vi "Initialize.vi"(8 "error in (no error)":errorcluster, 10 "Pixel Mode (0:Optical)":u16(ring) items=["Optical ", "All Pixels"], 11 "VISA resource name":refnum<visa-resource-name>) -> (0 "error out":errorcluster, 3 "VISA resource name out":refnum<visa-resource-name>)   [LabVIEW 2019, in "Ocean Optics 2000 4000.lvlib"]
doc: "Establishes communication with the instrument and optionally performs an instrument identification query and/or an instrument reset. It also places the instrument in a default state needed for other instrument driver operations. Therefore, call this VI before calling other instrument driver VIs for this instrument. Generally, you need to call the Initialize VI only once at the beginning of an application."
uses:
  Ocean Optics 2000 4000.lvlib
panel:
  # "(c) 2009-2016 National Instruments.  ALL RIGHTS RESERVED."
  # "Before using this driver:\n    * Go to Program Files >>National Instruments >>LabVIEW >> \n       instr.lib>> Ocean Optics 2000 4000>>VISA_USB\n    * Select the folder for the model of instrument you are using.\n    * For Windows Vista, use the INF file with _vista in the file name\n      (eg.Ocean Optics USB4000_vista.inf). For XP, use the other INF file.\n    * To install, right click and select Install.\n    * NI MAX should be able to detect this instrument after installing the \n      INF file."
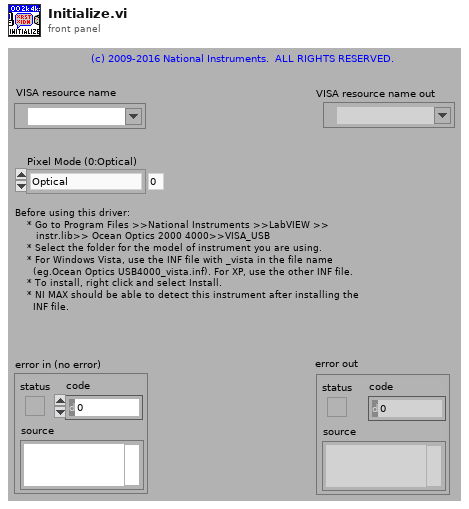
[diagram p1: front panel]
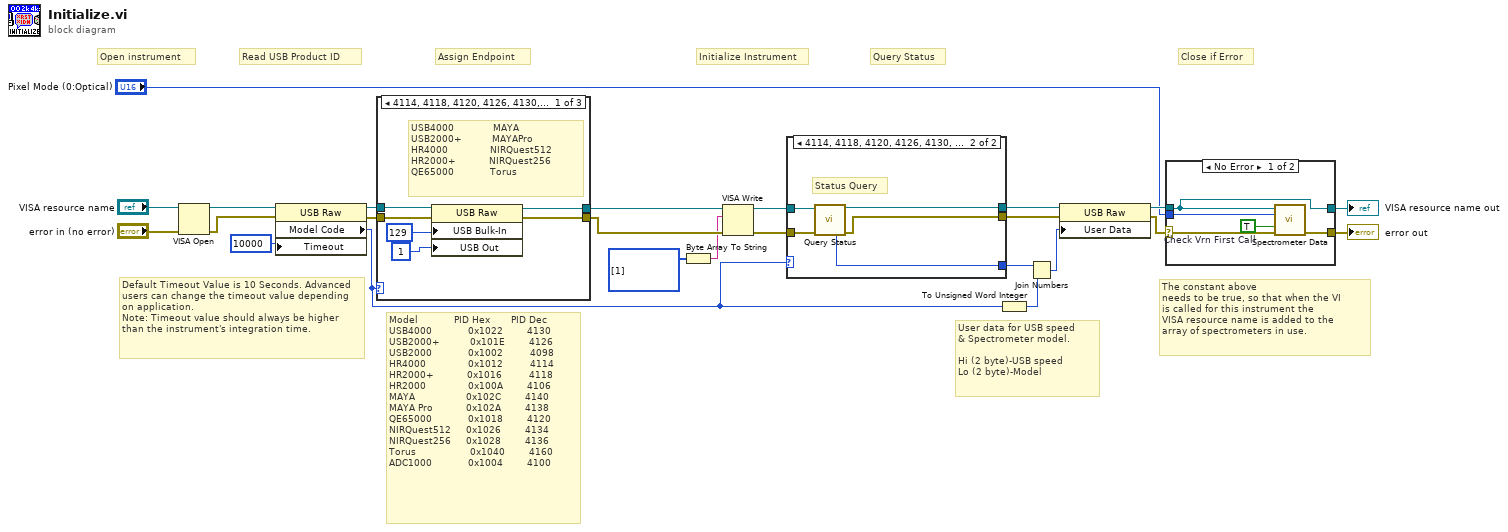
[diagram p0: block diagram]
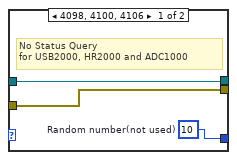
[diagram p2: hidden frame]
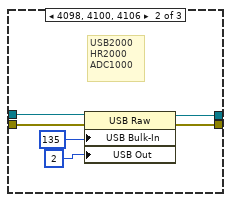
[diagram p3: hidden frame]
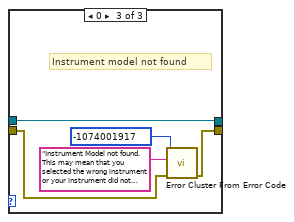
[diagram p4: hidden frame]
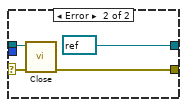
[diagram p5: hidden frame]
diagram:
  # "The constant above\nneeds to be true, so that when the VI \nis called for this instrument the \nVISA resource name is added to the \narray of spectrometers in use."
  # "Default Timeout Value is 10 Seconds. Advanced users can change the timeout value depending on application.\nNote: Timeout value should always be higher than the instrument's integration time."
  # "Model            PID Hex       PID Dec \nUSB4000            0x1022        4130 \nUSB2000+          0x101E        4126 \nUSB2000            0x1002         4098\nHR4000              0x1012         4114\nHR2000+           0x1016         4118\nHR2000              0x100A        4106\nMAYA                 0x102C        4140\nMAYA Pro           0x102A        4138\nQE65000            0x1018        4120\nNIRQuest512     0x1026        4134\nNIRQuest256     0x1028        4136\nTorus                  0x1040        4160\nADC1000            0x1004        4100"
  # "Read USB Product ID"
  # "Assign Endpoint"
  # "User data for USB speed \n& Spectrometer model. \n\nHi (2 byte)-USB speed\nLo (2 byte)-Model"
  # "Initialize Instrument"
  # "Query Status"
  # "Close if Error"
  # "Open instrument"
  n1 = VISA Open(error in (no error)="error in (no error)", VISA resource name="VISA resource name") -> (VISA resource name=w10:refnum<visa-resource-name>, error out=w9:errorcluster)  [unwired: 3 out]
  n2 = property class="USB Raw"(reference=w10, error in=w9, "Timeout"=u32 10000 ("General Settings:Timeout Value")) -> (reference out=w8:refnum<visa-resource-name>, error out=w7:errorcluster, "Model Code"=w3:u16)
  n3 = case shown="4114, 4118, 4120, 4126, 4130, 4134, 4136, 4138, 4140, 4160, Default" w3 {
    tunnel: [w30 w32 w41] -> w21
    tunnel: [w29 w31 w40] -> w20
    tunnel: w8 -> [w28 w34 w41]
    tunnel: w7 -> [w27 w33 w37]
    frame 4114, 4118, 4120, 4126, 4130, 4134, 4136, 4138, 4140, 4160, Default {
      # "USB4000             MAYA\nUSB2000+          MAYAPro     \nHR4000              NIRQuest512\nHR2000+           NIRQuest256   \nQE65000            Torus"
      n4 = property class="USB Raw"(reference=w28, error in=w27, "USB Bulk-In"=i16 129 ("USB Settings:Bulk-In Pipe"), "USB Out"=i16 1 ("USB Settings:Bulk-In Pipe")) -> (reference out=w30:refnum<visa-resource-name>, error out=w29:errorcluster)
    }
    frame 4098, 4100, 4106 {
      # "USB2000\nHR2000\nADC1000"
      n5 = property class="USB Raw"(reference=w34, error in=w33, "USB Bulk-In"=i16 135 ("USB Settings:Bulk-In Pipe"), "USB Out"=i16 2 ("USB Settings:Bulk-In Pipe")) -> (reference out=w32:refnum<visa-resource-name>, error out=w31:errorcluster)
    }
    frame 0 {
      # "Instrument model not found"
      n6 = call <vilib>:"Error Cluster From Error Code.vi"("error in (no error)"=w37, "error message (\"\")"="Instrument Model not found.This may mean that you selected the wrong instrument or your instrument did not respond.  You may also be using a model that is not officially supported by this driver. " ("error message (\"\")"), "error code (0)"=-1074001917) -> ("error out"=w40:errorcluster)  [unwired: 1 in, 5 out]
    }
  }
  n7 = Byte Array To String(unsigned byte array=u8[] [1] ("write buffer (empty)")) -> (string=w18:string)
  n8 = VISA Write(VISA resource name=w21, write buffer=w18, error in (no error)=w20) -> (VISA resource name out=w16:refnum<visa-resource-name>, error out=w15:errorcluster)  [unwired: 1 out]
  n9 = case shown="4114, 4118, 4120, 4126, 4130, 4134, 4136, 4138, 4140, 4160, Default" w3 {
    tunnel: w16 -> [w44 w49]
    tunnel: w15 -> [w43 w48]
    tunnel: [w44 w47] -> w14
    tunnel: [w43 w46] -> w13
    tunnel: [w42 w45] -> w6
    frame 4098, 4100, 4106 {
      w42 = u16 10  # Random number(not used)
      # "No Status Query \nfor USB2000, HR2000 and ADC1000"
    }
    frame 4114, 4118, 4120, 4126, 4130, 4134, 4136, 4138, 4140, 4160, Default {
      # "Status Query"
      n10 = call "Query Status.vi"("VISA resource name"=w49, "error in (no error)"=w48) -> ("VISA resource name out"=w47:refnum<visa-resource-name>, "USB Speed"=w45:u16, "error out"=w46:errorcluster)  [unwired: 11 out]
    }
  }
  n11 = To Unsigned Word Integer(number=w3) -> (unsigned 16bit integer=w5:u16)
  n12 = Join Numbers(hi=w6, lo=w5) -> ((hi.lo)=w4:u32)
  n13 = property class="USB Raw"(reference=w14, error in=w13, "User Data"=w4) -> (reference out=w12:refnum<visa-resource-name>, error out=w11:errorcluster)
  n14 = case shown="No Error" w11 {
    selector: w11 -> [w54 w57]
    tunnel: [w52 refnum<visa-resource-name> refnum ("VISA resource name out")] -> w24
    tunnel: [w53 w58] -> w23
    tunnel: w12 -> [w52 w55]
    tunnel: "Pixel Mode (0:Optical)" -> [w51 _]
    frame No Error {
      w50 = TRUE  # Check Vrn First Call
      n15 = call "Spectrometer Data.vi"("VISA resource name"=w52, "Pixel Mode (0:Optical)"=w51, "Check Vrn First Call (False)"=w50, "error in (no error)"=w54) -> ("error out"=w53:errorcluster)  [unwired: 6 in, 5 out]
    }
    frame Error {
      n16 = call "Close.vi"("error in (no error)"=w57, "VISA resource name"=w55) -> ("error out"=w58:errorcluster)  [unwired: 9 out]
    }
  }
  "VISA resource name out" <- w24
  "error out" <- w23
